vi "Async Stream ReadDI.vi"(8 "error in (no error)":errorcluster, 11 "DIOSessions In":T1) -> (0 "error out":errorcluster)   [LabVIEW 2019]
uses:
  Types/DIOSessions.ctl
  Types/DISession.ctl
  Types/DOSession.ctl
  Types/StreamReadDI.ctl
  Servers/ctet_dio/gRPC lvSupport/Server API/typeDefs/grpcId.ctl
  Servers/ctet_dio/ctet_dio Class/RPC Messages/measurementservice_ErrorOut/measurementservice_ErrorOut_Data.ctl
  Servers/ctet_dio/ctet_dio Class/RPC Messages/measurementservice_ReadDIResponse/measurementservice_ReadDIResponse_Data.ctl
  <vilib>/DAQmx/read.llb/DAQmx Read (Digital 1D Bool 1Chan 1Samp).vi
  <vilib>/DAQmx/read.llb/DAQmx Read (Digital 1D Bool NChan 1Samp 1Line).vi
  <vilib>/DAQmx/miscellaneous.llb/DAQmx Fill In Error Info.vi
  Servers/ctet_dio/ctet_dio Class/ctet_dio.lvclass
  Servers/ctet_dio/gRPC lvSupport/gprc-lvsupport.lvlib
  ctet_dio_User Library.lvlib
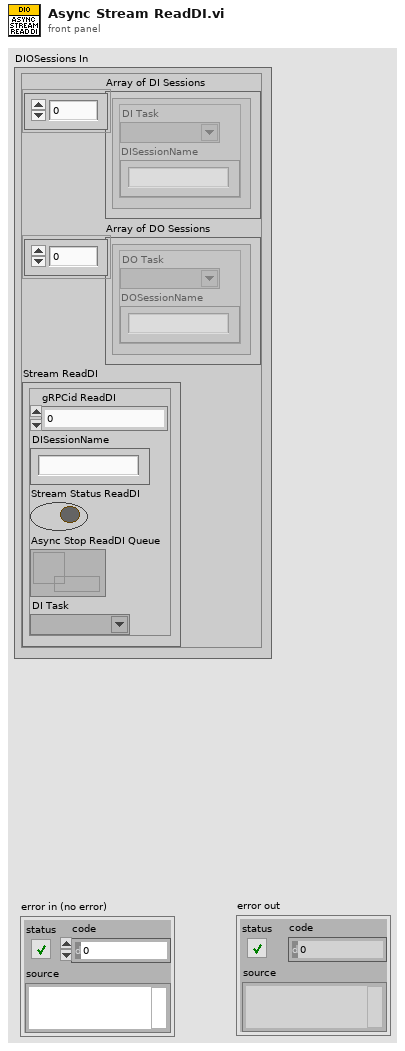
[diagram p1: front panel]
types:
  T1 = typedef "ctet_dio_User Library.lvlib/DIOSessions.ctl" = cluster{"Array of DI Sessions":T2[], "Array of DO Sessions":T3[], "Stream ReadDI":T4}
  T2 = typedef "ctet_dio_User Library.lvlib/DISession.ctl" = cluster{"DI Task":refnum<k21>, "DISessionName":string}
  T3 = typedef "ctet_dio_User Library.lvlib/DOSession.ctl" = cluster{"DO Task":refnum<k21>, "DOSessionName":string}
  T4 = typedef "ctet_dio_User Library.lvlib/StreamReadDI.ctl" = cluster{"gRPCid ReadDI":T5, "DISessionName":string, "Stream Status ReadDI":bool, "Async Stop ReadDI Queue":refnum<queue>, "DI Task":refnum<k21>}
  T5 = typedef "ctet_dio.lvlib/gprc-lvsupport.lvlib/grpcId.ctl" = u64
  T6 = typedef "ctet_dio.lvlib/ctet_dio.lvclass/measurementservice_ReadDIResponse_Data.ctl" = cluster{"DISessionName":string, "DIData":bool[], "error":T7}
  T7 = typedef "ctet_dio.lvlib/ctet_dio.lvclass/measurementservice_ErrorOut_Data.ctl" = cluster{"errCode":i64, "errMessage":string}
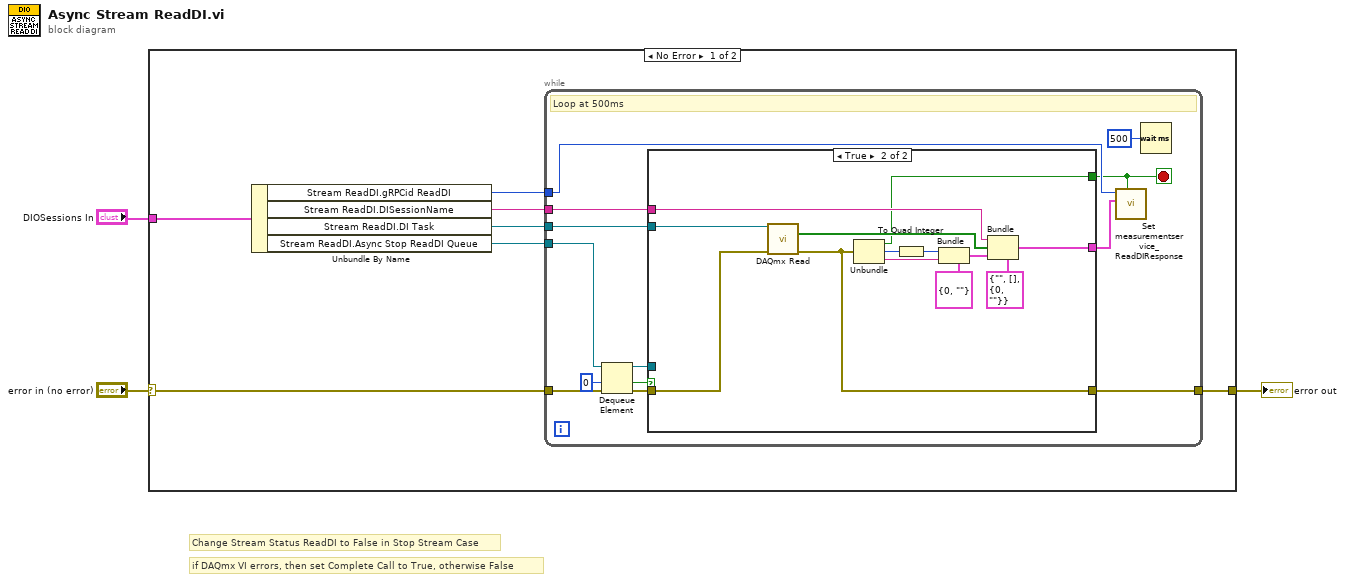
[diagram p0: block diagram]
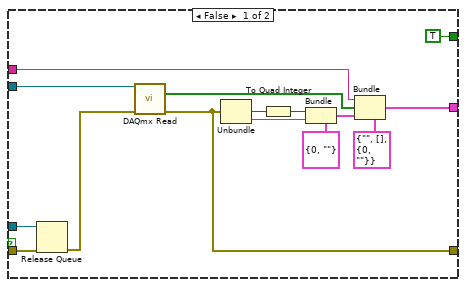
[diagram p2: hidden frame]
diagram:
  # "if DAQmx VI errors, then set Complete Call to True, otherwise False"
  # "Change Stream Status ReadDI to False in Stop Stream Case"
  n1 = case shown="No Error" "error in (no error)" {
    selector: "error in (no error)" -> [w7 w52]
    tunnel: [w4 w52] -> w3
    tunnel: "DIOSessions In" -> [w10 _]
    frame No Error {
      n2 = Unbundle By Name(w10) -> ("Stream ReadDI.gRPCid ReadDI"=w9:T5, "Stream ReadDI.DISessionName"=w6:string, "Stream ReadDI.DI Task"=w8:refnum<k21>, "Stream ReadDI.Async Stop ReadDI Queue"=w5:refnum<queue>)
      n3 = while {
        tunnel: w9 -> [w13]
        tunnel: w8 -> [w23]
        tunnel: w7 -> [w19]
        tunnel: w6 -> [w22]
        tunnel: w5 -> [w20]
        tunnel: [w12] -> w4
        stop <- w11 stop-if-true
        # "Loop at 500ms"
        n4 = Dequeue Element(queue=w20, timeout in ms (-1)=0, error in (no error)=w19) -> (queue out=w16:refnum<queue>, timed out?=w17:bool, error out=w15:errorcluster)  [unwired: 1 out]
        n5 = case shown="True" w17 {
          tunnel: w23 -> [w28 w44]
          tunnel: w22 -> [w24 w43]
          tunnel: w16 -> [w38 _]
          tunnel: w15 -> [w37 w40]
          tunnel: [w25 w42] -> w14
          tunnel: [TRUE ("Complete Call (T)") w39] -> w11
          tunnel: [w26 w41] -> w12
          frame False {
            n6 = Release Queue(queue=w38, error in (no error)=w37) -> (error out=w27:errorcluster)  [unwired: 1 in, 2 out]
            n7 = call-poly <vilib>:"DAQmx Read.vi"("task/channels in"=w28, "error in"=w27) -> ("data"=w29:bool[], "error out"=w26:errorcluster)  [unwired: 11 in, 1 out]
            n8 = Unbundle(w26) -> ("code"=w33:i32, "source"=w34:string)  [unwired: 1 out]
            n9 = To Quad Integer(1:w33) -> (0:w32:i64)
            n10 = Bundle(cluster=T7 {"errCode"=0, "errMessage"=""} ("error"), "errCode"=w32, "errMessage"=w34) -> (w30:T7)
            n11 = Bundle(cluster=T6 {"DISessionName"="", "DIData"=[], "error"={"errCode"=0, "errMessage"=""}} ("measurementservice_ReadDIResponse_Data"), "DISessionName"=w24, "DIData"=w29, "error"=w30) -> (w25:T6)
          }
          frame True {
            n12 = call-poly <vilib>:"DAQmx Read.vi"("task/channels in"=w44, "error in"=w40) -> ("data"=w45:bool[], "error out"=w41:errorcluster)  [unwired: 11 in, 1 out]
            n13 = Unbundle(w41) -> ("status"=w39:bool, "code"=w49:i32, "source"=w50:string)
            n14 = To Quad Integer(1:w49) -> (0:w48:i64)
            n15 = Bundle(cluster=T7 {"errCode"=0, "errMessage"=""} ("error"), "errCode"=w48, "errMessage"=w50) -> (w46:T7)
            n16 = Bundle(cluster=T6 {"DISessionName"="", "DIData"=[], "error"={"errCode"=0, "errMessage"=""}} ("measurementservice_ReadDIResponse_Data"), "DISessionName"=w43, "DIData"=w45, "error"=w46) -> (w42:T6)
          }
        }
        n17 = call "Set measurementservice_ReadDIResponse.vi"("Complete Call (T)"=w11, "Message Data"=w14, "gRPCid"=w13) -> ()  [unwired: 8 in, 1 out]
        n18 = Wait (ms)(milliseconds to wait=u32 500) -> ()  [unwired: 1 out]
      }
    }
    frame Error {
    }
  }
  "error out" <- w3
